vi "get Clock Free Running.vi"(11 "Clock Generator in":refnum<class "IO.lvclass">) -> (3 "Free Running":bool)   [LabVIEW 2021, in "IO.lvclass"]
uses:
  IO.lvclass
  IO.lvclass/IO.ctl
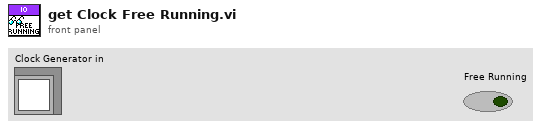
[diagram p1: front panel]
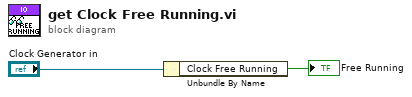
[diagram p0: block diagram]
diagram:
  n1 = Unbundle By Name("Clock Generator in") -> ("Clock Free Running"=→"Free Running":bool)
